vi "Tell Init Parent.vi"(7 "Actor in":refnum<class "Actor.lvclass">, 10 "Data":T1) -> (0 "Error out":errorcluster, 5 "Actor out":refnum<class "Actor.lvclass">)   [LabVIEW 2020, in "_Template.lvlib" / "Templates.lvlib" / "TEMPLATE jettl Msg.lvlib"]
uses:
  TEMPLATE jettl Msg.lvlib
  jettl/jettl/jettl.lvlib
  jettl/jettl/Actor/Actor.lvclass
  Data.ctl
panel:
  # "This front panel should not be manipulated."
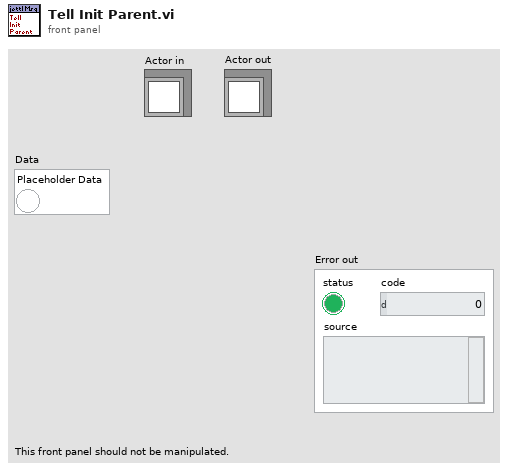
[diagram p1: front panel]
types:
  T1 = typedef "_Template.lvlib/Templates.lvlib/TEMPLATE jettl Msg.lvlib/Data.ctl" = cluster{"Placeholder Data":bool}
  T2 = typedef "jettl.lvlib/Msg.ctl" = cluster{"Msg":refnum<class "Msg.lvclass">, "Msg Contents":refnum<class "Msg Contents.lvclass">, "Teller":T3}
  T3 = typedef "jettl.lvlib/Teller.ctl" = cluster{"Unified Actor Alias":string, "Unified Actor Relation":T4, "Absolute Time":timestamp, "Relative Time":dbl}
  T4 = typedef "jettl.lvlib/Unified Actor Relation.ctl" = enum16{"Self", "Parent", "Child"}
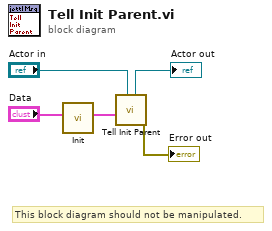
[diagram p0: block diagram]
diagram:
  # "This block diagram should not be manipulated."
  n1 = call "Init.vi"("Data"="Data") -> ("Msg"=w1:T2)  [unwired: 10 in]
  n2 = call "Tell Init Parent.vi"("Actor in"="Actor in", "Msg"=w1) -> ("Error out"=→"Error out":errorcluster, "Actor out"=→"Actor out":refnum<class "Actor.lvclass">)  [unwired: 8 in]
